vi "LoadImage_Names_more_robust.vi"(11 "Sample Image":path=path "E:/Temp/36ntATgel_20uM_10mMMg_20mMTris_4th/im__000015.tif") -> (1 "Paths":path[](array[path])=[path "E:/Temp/36ntATgel_20uM_10mMMg_20mMTris_4th/im__000003.tif", path "E:/Temp/36ntATgel_20uM_10mMMg_20mMTris_4th/im__000007.tif", path "E:/Temp/36ntATgel_20uM_10mMMg_20mMTris_4th/im__000011.tif", path "E:/Temp/36ntATgel_20uM_10mMMg_20mMTris_4th/im__000015.tif", path "E:/Temp/36ntATgel_20uM_10mMMg_20mMTris_4th/im__000019.tif", path "E:/Temp/36ntATgel_20uM_10mMMg_20mMTris_4th/im__000023.tif", path "E:/Temp/36ntATgel_20uM_10mMMg_20mMTris_4th/im__000027.tif", path "E:/Temp/36ntATgel_20uM_10mMMg_20mMTris_4th/im__000031.tif", path "E:/Temp/36ntATgel_20uM_10mMMg_20mMTris_4th/im__000035.tif", path "E:/Temp/36ntATgel_20uM_10mMMg_20mMTris_4th/im__000039.tif", path "E:/Temp/36ntATgel_20uM_10mMMg_20mMTris_4th/im__000043.tif", path "E:/Temp/36ntATgel_20uM_10mMMg_20mMTris_4th/im__000047.tif", path "E:/Temp/36ntATgel_20uM_10mMMg_20mMTris_4th/im__000051.tif", path "E:/Temp/36ntATgel_20uM_10mMMg_20mMTris_4th/im__000055.tif", path "E:/Temp/36ntATgel_20uM_10mMMg_20mMTris_4th/im__000059.tif", path "E:/Temp/36ntATgel_20uM_10mMMg_20mMTris_4th/im__000063.tif", path "E:/Temp/36ntATgel_20uM_10mMMg_20mMTris_4th/im__000067.tif", path "E:/Temp/36ntATgel_20uM_10mMMg_20mMTris_4th/im__000071.tif", path "E:/Temp/36ntATgel_20uM_10mMMg_20mMTris_4th/im__000075.tif", path "E:/Temp/36ntATgel_20uM_10mMMg_20mMTris_4th/im__000079.tif", path "E:/Temp/36ntATgel_20uM_10mMMg_20mMTris_4th/im__000083.tif", path "E:/Temp/36ntATgel_20uM_10mMMg_20mMTris_4th/im__000087.tif", path "E:/Temp/36ntATgel_20uM_10mMMg_20mMTris_4th/im__000091.tif", path "E:/Temp/36ntATgel_20uM_10mMMg_20mMTris_4th/im__000095.tif", path "E:/Temp/36ntATgel_20uM_10mMMg_20mMTris_4th/im__000099.tif", path "E:/Temp/36ntATgel_20uM_10mMMg_20mMTris_4th/im__000103.tif", path "E:/Temp/36ntATgel_20uM_10mMMg_20mMTris_4th/im__000107.tif", path "E:/Temp/36ntATgel_20uM_10mMMg_20mMTris_4th/im__000111.tif", path "E:/Temp/36ntATgel_20uM_10mMMg_20mMTris_4th/im__000115.tif", path "E:/Temp/36ntATgel_20uM_10mMMg_20mMTris_4th/im__000119.tif", path "E:/Temp/36ntATgel_20uM_10mMMg_20mMTris_4th/im__000123.tif", path "E:/Temp/36ntATgel_20uM_10mMMg_20mMTris_4th/im__000127.tif", path "E:/Temp/36ntATgel_20uM_10mMMg_20mMTris_4th/im__000131.tif", path "E:/Temp/36ntATgel_20uM_10mMMg_20mMTris_4th/im__000135.tif", path "E:/Temp/36ntATgel_20uM_10mMMg_20mMTris_4th/im__000139.tif", path "E:/Temp/36ntATgel_20uM_10mMMg_20mMTris_4th/im__000143.tif", path "E:/Temp/36ntATgel_20uM_10mMMg_20mMTris_4th/im__000147.tif", path "E:/Temp/36ntATgel_20uM_10mMMg_20mMTris_4th/im__000151.tif", path "E:/Temp/36ntATgel_20uM_10mMMg_20mMTris_4th/im__000155.tif", path "E:/Temp/36ntATgel_20uM_10mMMg_20mMTris_4th/im__000159.tif", path "E:/Temp/36ntATgel_20uM_10mMMg_20mMTris_4th/im__000163.tif", path "E:/Temp/36ntATgel_20uM_10mMMg_20mMTris_4th/im__000167.tif", path "E:/Temp/36ntATgel_20uM_10mMMg_20mMTris_4th/im__000171.tif", path "E:/Temp/36ntATgel_20uM_10mMMg_20mMTris_4th/im__000175.tif", path "E:/Temp/36ntATgel_20uM_10mMMg_20mMTris_4th/im__000179.tif", path "E:/Temp/36ntATgel_20uM_10mMMg_20mMTris_4th/im__000183.tif", path "E:/Temp/36ntATgel_20uM_10mMMg_20mMTris_4th/im__000187.tif", path "E:/Temp/36ntATgel_20uM_10mMMg_20mMTris_4th/im__000191.tif", path "E:/Temp/36ntATgel_20uM_10mMMg_20mMTris_4th/im__000195.tif", path "E:/Temp/36ntATgel_20uM_10mMMg_20mMTris_4th/im__000199.tif", path "E:/Temp/36ntATgel_20uM_10mMMg_20mMTris_4th/im__000203.tif", path "E:/Temp/36ntATgel_20uM_10mMMg_20mMTris_4th/im__000207.tif", path "E:/Temp/36ntATgel_20uM_10mMMg_20mMTris_4th/im__000211.tif", path "E:/Temp/36ntATgel_20uM_10mMMg_20mMTris_4th/im__000215.tif", path "E:/Temp/36ntATgel_20uM_10mMMg_20mMTris_4th/im__000219.tif", path "E:/Temp/36ntATgel_20uM_10mMMg_20mMTris_4th/im__000223.tif", path "E:/Temp/36ntATgel_20uM_10mMMg_20mMTris_4th/im__000227.tif", path "E:/Temp/36ntATgel_20uM_10mMMg_20mMTris_4th/im__000231.tif", path "E:/Temp/36ntATgel_20uM_10mMMg_20mMTris_4th/im__000235.tif", path "E:/Temp/36ntATgel_20uM_10mMMg_20mMTris_4th/im__000239.tif", path "E:/Temp/36ntATgel_20uM_10mMMg_20mMTris_4th/im__000243.tif", path "E:/Temp/36ntATgel_20uM_10mMMg_20mMTris_4th/im__000247.tif", path "E:/Temp/36ntATgel_20uM_10mMMg_20mMTris_4th/im__000251.tif", path "E:/Temp/36ntATgel_20uM_10mMMg_20mMTris_4th/im__000255.tif", path "E:/Temp/36ntATgel_20uM_10mMMg_20mMTris_4th/im__000259.tif", path "E:/Temp/36ntATgel_20uM_10mMMg_20mMTris_4th/im__000263.tif", path "E:/Temp/36ntATgel_20uM_10mMMg_20mMTris_4th/im__000267.tif", path "E:/Temp/36ntATgel_20uM_10mMMg_20mMTris_4th/im__000271.tif", path "E:/Temp/36ntATgel_20uM_10mMMg_20mMTris_4th/im__000275.tif", path "E:/Temp/36ntATgel_20uM_10mMMg_20mMTris_4th/im__000279.tif", path "E:/Temp/36ntATgel_20uM_10mMMg_20mMTris_4th/im__000283.tif", path "E:/Temp/36ntATgel_20uM_10mMMg_20mMTris_4th/im__000287.tif", path "E:/Temp/36ntATgel_20uM_10mMMg_20mMTris_4th/im__000291.tif", path "E:/Temp/36ntATgel_20uM_10mMMg_20mMTris_4th/im__000295.tif", path "E:/Temp/36ntATgel_20uM_10mMMg_20mMTris_4th/im__000299.tif", path "E:/Temp/36ntATgel_20uM_10mMMg_20mMTris_4th/im__000303.tif", path "E:/Temp/36ntATgel_20uM_10mMMg_20mMTris_4th/im__000307.tif", path "E:/Temp/36ntATgel_20uM_10mMMg_20mMTris_4th/im__000311.tif", path "E:/Temp/36ntATgel_20uM_10mMMg_20mMTris_4th/im__000315.tif", path "E:/Temp/36ntATgel_20uM_10mMMg_20mMTris_4th/im__000319.tif", path "E:/Temp/36ntATgel_20uM_10mMMg_20mMTris_4th/im__000323.tif", path "E:/Temp/36ntATgel_20uM_10mMMg_20mMTris_4th/im__000327.tif", path "E:/Temp/36ntATgel_20uM_10mMMg_20mMTris_4th/im__000331.tif", path "E:/Temp/36ntATgel_20uM_10mMMg_20mMTris_4th/im__000335.tif", path "E:/Temp/36ntATgel_20uM_10mMMg_20mMTris_4th/im__000339.tif", path "E:/Temp/36ntATgel_20uM_10mMMg_20mMTris_4th/im__000343.tif", path "E:/Temp/36ntATgel_20uM_10mMMg_20mMTris_4th/im__000347.tif", path "E:/Temp/36ntATgel_20uM_10mMMg_20mMTris_4th/im__000351.tif", path "E:/Temp/36ntATgel_20uM_10mMMg_20mMTris_4th/im__000355.tif", path "E:/Temp/36ntATgel_20uM_10mMMg_20mMTris_4th/im__000359.tif", path "E:/Temp/36ntATgel_20uM_10mMMg_20mMTris_4th/im__000363.tif", path "E:/Temp/36ntATgel_20uM_10mMMg_20mMTris_4th/im__000367.tif", path "E:/Temp/36ntATgel_20uM_10mMMg_20mMTris_4th/im__000371.tif", path "E:/Temp/36ntATgel_20uM_10mMMg_20mMTris_4th/im__000375.tif", path "E:/Temp/36ntATgel_20uM_10mMMg_20mMTris_4th/im__000379.tif", path "E:/Temp/36ntATgel_20uM_10mMMg_20mMTris_4th/im__000383.tif", path "E:/Temp/36ntATgel_20uM_10mMMg_20mMTris_4th/im__000387.tif", path "E:/Temp/36ntATgel_20uM_10mMMg_20mMTris_4th/im__000391.tif", path "E:/Temp/36ntATgel_20uM_10mMMg_20mMTris_4th/im__000395.tif", path "E:/Temp/36ntATgel_20uM_10mMMg_20mMTris_4th/im__000399.tif", path "E:/Temp/36ntATgel_20uM_10mMMg_20mMTris_4th/im__000403.tif", path "E:/Temp/36ntATgel_20uM_10mMMg_20mMTris_4th/im__000407.tif", path "E:/Temp/36ntATgel_20uM_10mMMg_20mMTris_4th/im__000411.tif", path "E:/Temp/36ntATgel_20uM_10mMMg_20mMTris_4th/im__000415.tif", path "E:/Temp/36ntATgel_20uM_10mMMg_20mMTris_4th/im__000419.tif", path "E:/Temp/36ntATgel_20uM_10mMMg_20mMTris_4th/im__000423.tif", path "E:/Temp/36ntATgel_20uM_10mMMg_20mMTris_4th/im__000427.tif", path "E:/Temp/36ntATgel_20uM_10mMMg_20mMTris_4th/im__000431.tif", path "E:/Temp/36ntATgel_20uM_10mMMg_20mMTris_4th/im__000435.tif", path "E:/Temp/36ntATgel_20uM_10mMMg_20mMTris_4th/im__000439.tif", path "E:/Temp/36ntATgel_20uM_10mMMg_20mMTris_4th/im__000443.tif", path "E:/Temp/36ntATgel_20uM_10mMMg_20mMTris_4th/im__000447.tif", path "E:/Temp/36ntATgel_20uM_10mMMg_20mMTris_4th/im__000451.tif", path "E:/Temp/36ntATgel_20uM_10mMMg_20mMTris_4th/im__000455.tif", path "E:/Temp/36ntATgel_20uM_10mMMg_20mMTris_4th/im__000459.tif", path "E:/Temp/36ntATgel_20uM_10mMMg_20mMTris_4th/im__000463.tif", path "E:/Temp/36ntATgel_20uM_10mMMg_20mMTris_4th/im__000467.tif", path "E:/Temp/36ntATgel_20uM_10mMMg_20mMTris_4th/im__000471.tif", path "E:/Temp/36ntATgel_20uM_10mMMg_20mMTris_4th/im__000475.tif", path "E:/Temp/36ntATgel_20uM_10mMMg_20mMTris_4th/im__000479.tif", path "E:/Temp/36ntATgel_20uM_10mMMg_20mMTris_4th/im__000483.tif", path "E:/Temp/36ntATgel_20uM_10mMMg_20mMTris_4th/im__000487.tif", path "E:/Temp/36ntATgel_20uM_10mMMg_20mMTris_4th/im__000491.tif", path "E:/Temp/36ntATgel_20uM_10mMMg_20mMTris_4th/im__000495.tif", path "E:/Temp/36ntATgel_20uM_10mMMg_20mMTris_4th/im__000499.tif", path "E:/Temp/36ntATgel_20uM_10mMMg_20mMTris_4th/im__000503.tif", path "E:/Temp/36ntATgel_20uM_10mMMg_20mMTris_4th/im__000507.tif", path "E:/Temp/36ntATgel_20uM_10mMMg_20mMTris_4th/im__000511.tif", path "E:/Temp/36ntATgel_20uM_10mMMg_20mMTris_4th/im__000515.tif", path "E:/Temp/36ntATgel_20uM_10mMMg_20mMTris_4th/im__000519.tif", path "E:/Temp/36ntATgel_20uM_10mMMg_20mMTris_4th/im__000523.tif", path "E:/Temp/36ntATgel_20uM_10mMMg_20mMTris_4th/im__000527.tif", path "E:/Temp/36ntATgel_20uM_10mMMg_20mMTris_4th/im__000531.tif", path "E:/Temp/36ntATgel_20uM_10mMMg_20mMTris_4th/im__000535.tif", path "E:/Temp/36ntATgel_20uM_10mMMg_20mMTris_4th/im__000539.tif", path "E:/Temp/36ntATgel_20uM_10mMMg_20mMTris_4th/im__000543.tif", path "E:/Temp/36ntATgel_20uM_10mMMg_20mMTris_4th/im__000547.tif", path "E:/Temp/36ntATgel_20uM_10mMMg_20mMTris_4th/im__000551.tif", path "E:/Temp/36ntATgel_20uM_10mMMg_20mMTris_4th/im__000555.tif", path "E:/Temp/36ntATgel_20uM_10mMMg_20mMTris_4th/im__000559.tif", path "E:/Temp/36ntATgel_20uM_10mMMg_20mMTris_4th/im__000563.tif", path "E:/Temp/36ntATgel_20uM_10mMMg_20mMTris_4th/im__000567.tif", path "E:/Temp/36ntATgel_20uM_10mMMg_20mMTris_4th/im__000571.tif", path "E:/Temp/36ntATgel_20uM_10mMMg_20mMTris_4th/im__000575.tif", path "E:/Temp/36ntATgel_20uM_10mMMg_20mMTris_4th/im__000579.tif", path "E:/Temp/36ntATgel_20uM_10mMMg_20mMTris_4th/im__000583.tif", path "E:/Temp/36ntATgel_20uM_10mMMg_20mMTris_4th/im__000587.tif", path "E:/Temp/36ntATgel_20uM_10mMMg_20mMTris_4th/im__000591.tif", path "E:/Temp/36ntATgel_20uM_10mMMg_20mMTris_4th/im__000595.tif", path "E:/Temp/36ntATgel_20uM_10mMMg_20mMTris_4th/im__000599.tif", path "E:/Temp/36ntATgel_20uM_10mMMg_20mMTris_4th/im__000603.tif", path "E:/Temp/36ntATgel_20uM_10mMMg_20mMTris_4th/im__000607.tif", path "E:/Temp/36ntATgel_20uM_10mMMg_20mMTris_4th/im__000611.tif", path "E:/Temp/36ntATgel_20uM_10mMMg_20mMTris_4th/im__000615.tif", path "E:/Temp/36ntATgel_20uM_10mMMg_20mMTris_4th/im__000619.tif", path "E:/Temp/36ntATgel_20uM_10mMMg_20mMTris_4th/im__000623.tif", path "E:/Temp/36ntATgel_20uM_10mMMg_20mMTris_4th/im__000627.tif", path "E:/Temp/36ntATgel_20uM_10mMMg_20mMTris_4th/im__000631.tif", path "E:/Temp/36ntATgel_20uM_10mMMg_20mMTris_4th/im__000635.tif", path "E:/Temp/36ntATgel_20uM_10mMMg_20mMTris_4th/im__000639.tif", path "E:/Temp/36ntATgel_20uM_10mMMg_20mMTris_4th/im__000643.tif", path "E:/Temp/36ntATgel_20uM_10mMMg_20mMTris_4th/im__000647.tif", path "E:/Temp/36ntATgel_20uM_10mMMg_20mMTris_4th/im__000651.tif", path "E:/Temp/36ntATgel_20uM_10mMMg_20mMTris_4th/im__000655.tif", path "E:/Temp/36ntATgel_20uM_10mMMg_20mMTris_4th/im__000659.tif", path "E:/Temp/36ntATgel_20uM_10mMMg_20mMTris_4th/im__000663.tif", path "E:/Temp/36ntATgel_20uM_10mMMg_20mMTris_4th/im__000667.tif", path "E:/Temp/36ntATgel_20uM_10mMMg_20mMTris_4th/im__000671.tif", path "E:/Temp/36ntATgel_20uM_10mMMg_20mMTris_4th/im__000675.tif", path "E:/Temp/36ntATgel_20uM_10mMMg_20mMTris_4th/im__000679.tif", path "E:/Temp/36ntATgel_20uM_10mMMg_20mMTris_4th/im__000683.tif", path "E:/Temp/36ntATgel_20uM_10mMMg_20mMTris_4th/im__000687.tif", path "E:/Temp/36ntATgel_20uM_10mMMg_20mMTris_4th/im__000691.tif", path "E:/Temp/36ntATgel_20uM_10mMMg_20mMTris_4th/im__000695.tif", path "E:/Temp/36ntATgel_20uM_10mMMg_20mMTris_4th/im__000699.tif", path "E:/Temp/36ntATgel_20uM_10mMMg_20mMTris_4th/im__000703.tif", path "E:/Temp/36ntATgel_20uM_10mMMg_20mMTris_4th/im__000707.tif", path "E:/Temp/36ntATgel_20uM_10mMMg_20mMTris_4th/im__000711.tif", path "E:/Temp/36ntATgel_20uM_10mMMg_20mMTris_4th/im__000715.tif", path "E:/Temp/36ntATgel_20uM_10mMMg_20mMTris_4th/im__000719.tif", path "E:/Temp/36ntATgel_20uM_10mMMg_20mMTris_4th/im__000723.tif", path "E:/Temp/36ntATgel_20uM_10mMMg_20mMTris_4th/im__000727.tif", path "E:/Temp/36ntATgel_20uM_10mMMg_20mMTris_4th/im__000731.tif", path "E:/Temp/36ntATgel_20uM_10mMMg_20mMTris_4th/im__000735.tif", path "E:/Temp/36ntATgel_20uM_10mMMg_20mMTris_4th/im__000739.tif", path "E:/Temp/36ntATgel_20uM_10mMMg_20mMTris_4th/im__000743.tif", path "E:/Temp/36ntATgel_20uM_10mMMg_20mMTris_4th/im__000747.tif", path "E:/Temp/36ntATgel_20uM_10mMMg_20mMTris_4th/im__000751.tif", path "E:/Temp/36ntATgel_20uM_10mMMg_20mMTris_4th/im__000755.tif", path "E:/Temp/36ntATgel_20uM_10mMMg_20mMTris_4th/im__000759.tif", path "E:/Temp/36ntATgel_20uM_10mMMg_20mMTris_4th/im__000763.tif", path "E:/Temp/36ntATgel_20uM_10mMMg_20mMTris_4th/im__000767.tif", path "E:/Temp/36ntATgel_20uM_10mMMg_20mMTris_4th/im__000771.tif", path "E:/Temp/36ntATgel_20uM_10mMMg_20mMTris_4th/im__000775.tif", path "E:/Temp/36ntATgel_20uM_10mMMg_20mMTris_4th/im__000779.tif", path "E:/Temp/36ntATgel_20uM_10mMMg_20mMTris_4th/im__000783.tif", path "E:/Temp/36ntATgel_20uM_10mMMg_20mMTris_4th/im__000787.tif", path "E:/Temp/36ntATgel_20uM_10mMMg_20mMTris_4th/im__000791.tif", path "E:/Temp/36ntATgel_20uM_10mMMg_20mMTris_4th/im__000795.tif", path "E:/Temp/36ntATgel_20uM_10mMMg_20mMTris_4th/im__000799.tif", path "E:/Temp/36ntATgel_20uM_10mMMg_20mMTris_4th/im__000803.tif", path "E:/Temp/36ntATgel_20uM_10mMMg_20mMTris_4th/im__000807.tif", path "E:/Temp/36ntATgel_20uM_10mMMg_20mMTris_4th/im__000811.tif", path "E:/Temp/36ntATgel_20uM_10mMMg_20mMTris_4th/im__000815.tif", path "E:/Temp/36ntATgel_20uM_10mMMg_20mMTris_4th/im__000819.tif", path "E:/Temp/36ntATgel_20uM_10mMMg_20mMTris_4th/im__000823.tif", path "E:/Temp/36ntATgel_20uM_10mMMg_20mMTris_4th/im__000827.tif", path "E:/Temp/36ntATgel_20uM_10mMMg_20mMTris_4th/im__000831.tif", path "E:/Temp/36ntATgel_20uM_10mMMg_20mMTris_4th/im__000835.tif", path "E:/Temp/36ntATgel_20uM_10mMMg_20mMTris_4th/im__000839.tif", path "E:/Temp/36ntATgel_20uM_10mMMg_20mMTris_4th/im__000843.tif", path "E:/Temp/36ntATgel_20uM_10mMMg_20mMTris_4th/im__000847.tif", path "E:/Temp/36ntATgel_20uM_10mMMg_20mMTris_4th/im__000851.tif", path "E:/Temp/36ntATgel_20uM_10mMMg_20mMTris_4th/im__000855.tif", path "E:/Temp/36ntATgel_20uM_10mMMg_20mMTris_4th/im__000859.tif", path "E:/Temp/36ntATgel_20uM_10mMMg_20mMTris_4th/im__000863.tif", path "E:/Temp/36ntATgel_20uM_10mMMg_20mMTris_4th/im__000867.tif", path "E:/Temp/36ntATgel_20uM_10mMMg_20mMTris_4th/im__000871.tif", path "E:/Temp/36ntATgel_20uM_10mMMg_20mMTris_4th/im__000875.tif", path "E:/Temp/36ntATgel_20uM_10mMMg_20mMTris_4th/im__000879.tif", path "E:/Temp/36ntATgel_20uM_10mMMg_20mMTris_4th/im__000883.tif", path "E:/Temp/36ntATgel_20uM_10mMMg_20mMTris_4th/im__000887.tif", path "E:/Temp/36ntATgel_20uM_10mMMg_20mMTris_4th/im__000891.tif", path "E:/Temp/36ntATgel_20uM_10mMMg_20mMTris_4th/im__000895.tif", path "E:/Temp/36ntATgel_20uM_10mMMg_20mMTris_4th/im__000899.tif", path "E:/Temp/36ntATgel_20uM_10mMMg_20mMTris_4th/im__000903.tif", path "E:/Temp/36ntATgel_20uM_10mMMg_20mMTris_4th/im__000907.tif", path "E:/Temp/36ntATgel_20uM_10mMMg_20mMTris_4th/im__000911.tif", path "E:/Temp/36ntATgel_20uM_10mMMg_20mMTris_4th/im__000915.tif", path "E:/Temp/36ntATgel_20uM_10mMMg_20mMTris_4th/im__000919.tif", path "E:/Temp/36ntATgel_20uM_10mMMg_20mMTris_4th/im__000923.tif", path "E:/Temp/36ntATgel_20uM_10mMMg_20mMTris_4th/im__000927.tif", path "E:/Temp/36ntATgel_20uM_10mMMg_20mMTris_4th/im__000931.tif", path "E:/Temp/36ntATgel_20uM_10mMMg_20mMTris_4th/im__000935.tif", path "E:/Temp/36ntATgel_20uM_10mMMg_20mMTris_4th/im__000939.tif", path "E:/Temp/36ntATgel_20uM_10mMMg_20mMTris_4th/im__000943.tif", path "E:/Temp/36ntATgel_20uM_10mMMg_20mMTris_4th/im__000947.tif", path "E:/Temp/36ntATgel_20uM_10mMMg_20mMTris_4th/im__000951.tif", path "E:/Temp/36ntATgel_20uM_10mMMg_20mMTris_4th/im__000955.tif", path "E:/Temp/36ntATgel_20uM_10mMMg_20mMTris_4th/im__000959.tif", path "E:/Temp/36ntATgel_20uM_10mMMg_20mMTris_4th/im__000963.tif", path "E:/Temp/36ntATgel_20uM_10mMMg_20mMTris_4th/im__000967.tif", path "E:/Temp/36ntATgel_20uM_10mMMg_20mMTris_4th/im__000971.tif", path "E:/Temp/36ntATgel_20uM_10mMMg_20mMTris_4th/im__000975.tif", path "E:/Temp/36ntATgel_20uM_10mMMg_20mMTris_4th/im__000979.tif", path "E:/Temp/36ntATgel_20uM_10mMMg_20mMTris_4th/im__000983.tif", path "E:/Temp/36ntATgel_20uM_10mMMg_20mMTris_4th/im__000987.tif", path "E:/Temp/36ntATgel_20uM_10mMMg_20mMTris_4th/im__000991.tif", path "E:/Temp/36ntATgel_20uM_10mMMg_20mMTris_4th/im__000995.tif", path "E:/Temp/36ntATgel_20uM_10mMMg_20mMTris_4th/im__000999.tif", path "E:/Temp/36ntATgel_20uM_10mMMg_20mMTris_4th/im__001003.tif", path "E:/Temp/36ntATgel_20uM_10mMMg_20mMTris_4th/im__001007.tif", path "E:/Temp/36ntATgel_20uM_10mMMg_20mMTris_4th/im__001011.tif", path "E:/Temp/36ntATgel_20uM_10mMMg_20mMTris_4th/im__001015.tif", path "E:/Temp/36ntATgel_20uM_10mMMg_20mMTris_4th/im__001019.tif", path "E:/Temp/36ntATgel_20uM_10mMMg_20mMTris_4th/im__001023.tif", path "E:/Temp/36ntATgel_20uM_10mMMg_20mMTris_4th/im__001027.tif", path "E:/Temp/36ntATgel_20uM_10mMMg_20mMTris_4th/im__001031.tif", path "E:/Temp/36ntATgel_20uM_10mMMg_20mMTris_4th/im__001035.tif", path "E:/Temp/36ntATgel_20uM_10mMMg_20mMTris_4th/im__001039.tif", path "E:/Temp/36ntATgel_20uM_10mMMg_20mMTris_4th/im__001043.tif", path "E:/Temp/36ntATgel_20uM_10mMMg_20mMTris_4th/im__001047.tif", path "E:/Temp/36ntATgel_20uM_10mMMg_20mMTris_4th/im__001051.tif", path "E:/Temp/36ntATgel_20uM_10mMMg_20mMTris_4th/im__001055.tif", path "E:/Temp/36ntATgel_20uM_10mMMg_20mMTris_4th/im__001059.tif", path "E:/Temp/36ntATgel_20uM_10mMMg_20mMTris_4th/im__001063.tif", path "E:/Temp/36ntATgel_20uM_10mMMg_20mMTris_4th/im__001067.tif", path "E:/Temp/36ntATgel_20uM_10mMMg_20mMTris_4th/im__001071.tif", path "E:/Temp/36ntATgel_20uM_10mMMg_20mMTris_4th/im__001075.tif", path "E:/Temp/36ntATgel_20uM_10mMMg_20mMTris_4th/im__001079.tif", path "E:/Temp/36ntATgel_20uM_10mMMg_20mMTris_4th/im__001083.tif", path "E:/Temp/36ntATgel_20uM_10mMMg_20mMTris_4th/im__001087.tif", path "E:/Temp/36ntATgel_20uM_10mMMg_20mMTris_4th/im__001091.tif", path "E:/Temp/36ntATgel_20uM_10mMMg_20mMTris_4th/im__001095.tif", path "E:/Temp/36ntATgel_20uM_10mMMg_20mMTris_4th/im__001099.tif", path "E:/Temp/36ntATgel_20uM_10mMMg_20mMTris_4th/im__001103.tif", path "E:/Temp/36ntATgel_20uM_10mMMg_20mMTris_4th/im__001107.tif", path "E:/Temp/36ntATgel_20uM_10mMMg_20mMTris_4th/im__001111.tif", path "E:/Temp/36ntATgel_20uM_10mMMg_20mMTris_4th/im__001115.tif", path "E:/Temp/36ntATgel_20uM_10mMMg_20mMTris_4th/im__001119.tif", path "E:/Temp/36ntATgel_20uM_10mMMg_20mMTris_4th/im__001123.tif", path "E:/Temp/36ntATgel_20uM_10mMMg_20mMTris_4th/im__001127.tif", path "E:/Temp/36ntATgel_20uM_10mMMg_20mMTris_4th/im__001131.tif", path "E:/Temp/36ntATgel_20uM_10mMMg_20mMTris_4th/im__001135.tif", path "E:/Temp/36ntATgel_20uM_10mMMg_20mMTris_4th/im__001139.tif", path "E:/Temp/36ntATgel_20uM_10mMMg_20mMTris_4th/im__001143.tif", path "E:/Temp/36ntATgel_20uM_10mMMg_20mMTris_4th/im__001147.tif", path "E:/Temp/36ntATgel_20uM_10mMMg_20mMTris_4th/im__001151.tif", path "E:/Temp/36ntATgel_20uM_10mMMg_20mMTris_4th/im__001155.tif", path "E:/Temp/36ntATgel_20uM_10mMMg_20mMTris_4th/im__001159.tif", path "E:/Temp/36ntATgel_20uM_10mMMg_20mMTris_4th/im__001163.tif", path "E:/Temp/36ntATgel_20uM_10mMMg_20mMTris_4th/im__001167.tif", path "E:/Temp/36ntATgel_20uM_10mMMg_20mMTris_4th/im__001171.tif", path "E:/Temp/36ntATgel_20uM_10mMMg_20mMTris_4th/im__001175.tif", path "E:/Temp/36ntATgel_20uM_10mMMg_20mMTris_4th/im__001179.tif", path "E:/Temp/36ntATgel_20uM_10mMMg_20mMTris_4th/im__001183.tif", path "E:/Temp/36ntATgel_20uM_10mMMg_20mMTris_4th/im__001187.tif", path "E:/Temp/36ntATgel_20uM_10mMMg_20mMTris_4th/im__001191.tif", path "E:/Temp/36ntATgel_20uM_10mMMg_20mMTris_4th/im__001195.tif", path "E:/Temp/36ntATgel_20uM_10mMMg_20mMTris_4th/im__001199.tif", path "E:/Temp/36ntATgel_20uM_10mMMg_20mMTris_4th/im__001203.tif", path "E:/Temp/36ntATgel_20uM_10mMMg_20mMTris_4th/im__001207.tif", path "E:/Temp/36ntATgel_20uM_10mMMg_20mMTris_4th/im__001211.tif", path "E:/Temp/36ntATgel_20uM_10mMMg_20mMTris_4th/im__001215.tif", path "E:/Temp/36ntATgel_20uM_10mMMg_20mMTris_4th/im__001219.tif", path "E:/Temp/36ntATgel_20uM_10mMMg_20mMTris_4th/im__001223.tif", path "E:/Temp/36ntATgel_20uM_10mMMg_20mMTris_4th/im__001227.tif", path "E:/Temp/36ntATgel_20uM_10mMMg_20mMTris_4th/im__001231.tif", path "E:/Temp/36ntATgel_20uM_10mMMg_20mMTris_4th/im__001235.tif", path "E:/Temp/36ntATgel_20uM_10mMMg_20mMTris_4th/im__001239.tif", path "E:/Temp/36ntATgel_20uM_10mMMg_20mMTris_4th/im__001243.tif", path "E:/Temp/36ntATgel_20uM_10mMMg_20mMTris_4th/im__001247.tif", path "E:/Temp/36ntATgel_20uM_10mMMg_20mMTris_4th/im__001251.tif", path "E:/Temp/36ntATgel_20uM_10mMMg_20mMTris_4th/im__001255.tif", path "E:/Temp/36ntATgel_20uM_10mMMg_20mMTris_4th/im__001259.tif", path "E:/Temp/36ntATgel_20uM_10mMMg_20mMTris_4th/im__001263.tif", path "E:/Temp/36ntATgel_20uM_10mMMg_20mMTris_4th/im__001267.tif", path "E:/Temp/36ntATgel_20uM_10mMMg_20mMTris_4th/im__001271.tif", path "E:/Temp/36ntATgel_20uM_10mMMg_20mMTris_4th/im__001275.tif", path "E:/Temp/36ntATgel_20uM_10mMMg_20mMTris_4th/im__001279.tif", path "E:/Temp/36ntATgel_20uM_10mMMg_20mMTris_4th/im__001283.tif", path "E:/Temp/36ntATgel_20uM_10mMMg_20mMTris_4th/im__001287.tif", path "E:/Temp/36ntATgel_20uM_10mMMg_20mMTris_4th/im__001291.tif", path "E:/Temp/36ntATgel_20uM_10mMMg_20mMTris_4th/im__001295.tif", path "E:/Temp/36ntATgel_20uM_10mMMg_20mMTris_4th/im__001299.tif", path "E:/Temp/36ntATgel_20uM_10mMMg_20mMTris_4th/im__001303.tif", path "E:/Temp/36ntATgel_20uM_10mMMg_20mMTris_4th/im__001307.tif", path "E:/Temp/36ntATgel_20uM_10mMMg_20mMTris_4th/im__001311.tif", path "E:/Temp/36ntATgel_20uM_10mMMg_20mMTris_4th/im__001315.tif", path "E:/Temp/36ntATgel_20uM_10mMMg_20mMTris_4th/im__001319.tif", path "E:/Temp/36ntATgel_20uM_10mMMg_20mMTris_4th/im__001323.tif", path "E:/Temp/36ntATgel_20uM_10mMMg_20mMTris_4th/im__001327.tif", path "E:/Temp/36ntATgel_20uM_10mMMg_20mMTris_4th/im__001331.tif", path "E:/Temp/36ntATgel_20uM_10mMMg_20mMTris_4th/im__001335.tif", path "E:/Temp/36ntATgel_20uM_10mMMg_20mMTris_4th/im__001339.tif", path "E:/Temp/36ntATgel_20uM_10mMMg_20mMTris_4th/im__001343.tif", path "E:/Temp/36ntATgel_20uM_10mMMg_20mMTris_4th/im__001347.tif", path "E:/Temp/36ntATgel_20uM_10mMMg_20mMTris_4th/im__001351.tif", path "E:/Temp/36ntATgel_20uM_10mMMg_20mMTris_4th/im__001355.tif", path "E:/Temp/36ntATgel_20uM_10mMMg_20mMTris_4th/im__001359.tif", path "E:/Temp/36ntATgel_20uM_10mMMg_20mMTris_4th/im__001363.tif", path "E:/Temp/36ntATgel_20uM_10mMMg_20mMTris_4th/im__001367.tif", path "E:/Temp/36ntATgel_20uM_10mMMg_20mMTris_4th/im__001371.tif", path "E:/Temp/36ntATgel_20uM_10mMMg_20mMTris_4th/im__001375.tif", path "E:/Temp/36ntATgel_20uM_10mMMg_20mMTris_4th/im__001379.tif", path "E:/Temp/36ntATgel_20uM_10mMMg_20mMTris_4th/im__001383.tif", path "E:/Temp/36ntATgel_20uM_10mMMg_20mMTris_4th/im__001387.tif", path "E:/Temp/36ntATgel_20uM_10mMMg_20mMTris_4th/im__001391.tif", path "E:/Temp/36ntATgel_20uM_10mMMg_20mMTris_4th/im__001395.tif", path "E:/Temp/36ntATgel_20uM_10mMMg_20mMTris_4th/im__001399.tif", path "E:/Temp/36ntATgel_20uM_10mMMg_20mMTris_4th/im__001403.tif", path "E:/Temp/36ntATgel_20uM_10mMMg_20mMTris_4th/im__001407.tif", path "E:/Temp/36ntATgel_20uM_10mMMg_20mMTris_4th/im__001411.tif", path "E:/Temp/36ntATgel_20uM_10mMMg_20mMTris_4th/im__001415.tif", path "E:/Temp/36ntATgel_20uM_10mMMg_20mMTris_4th/im__001419.tif", path "E:/Temp/36ntATgel_20uM_10mMMg_20mMTris_4th/im__001423.tif", path "E:/Temp/36ntATgel_20uM_10mMMg_20mMTris_4th/im__001427.tif", path "E:/Temp/36ntATgel_20uM_10mMMg_20mMTris_4th/im__001431.tif", path "E:/Temp/36ntATgel_20uM_10mMMg_20mMTris_4th/im__001435.tif", path "E:/Temp/36ntATgel_20uM_10mMMg_20mMTris_4th/im__001439.tif", path "E:/Temp/36ntATgel_20uM_10mMMg_20mMTris_4th/im__001443.tif", path "E:/Temp/36ntATgel_20uM_10mMMg_20mMTris_4th/im__001447.tif", path "E:/Temp/36ntATgel_20uM_10mMMg_20mMTris_4th/im__001451.tif", path "E:/Temp/36ntATgel_20uM_10mMMg_20mMTris_4th/im__001455.tif", path "E:/Temp/36ntATgel_20uM_10mMMg_20mMTris_4th/im__001459.tif", path "E:/Temp/36ntATgel_20uM_10mMMg_20mMTris_4th/im__001463.tif", path "E:/Temp/36ntATgel_20uM_10mMMg_20mMTris_4th/im__001467.tif", path "E:/Temp/36ntATgel_20uM_10mMMg_20mMTris_4th/im__001471.tif", path "E:/Temp/36ntATgel_20uM_10mMMg_20mMTris_4th/im__001475.tif", path "E:/Temp/36ntATgel_20uM_10mMMg_20mMTris_4th/im__001479.tif", path "E:/Temp/36ntATgel_20uM_10mMMg_20mMTris_4th/im__001483.tif", path "E:/Temp/36ntATgel_20uM_10mMMg_20mMTris_4th/im__001487.tif", path "E:/Temp/36ntATgel_20uM_10mMMg_20mMTris_4th/im__001491.tif", path "E:/Temp/36ntATgel_20uM_10mMMg_20mMTris_4th/im__001495.tif", path "E:/Temp/36ntATgel_20uM_10mMMg_20mMTris_4th/im__001499.tif", path "E:/Temp/36ntATgel_20uM_10mMMg_20mMTris_4th/im__001503.tif", path "E:/Temp/36ntATgel_20uM_10mMMg_20mMTris_4th/im__001507.tif", path "E:/Temp/36ntATgel_20uM_10mMMg_20mMTris_4th/im__001511.tif", path "E:/Temp/36ntATgel_20uM_10mMMg_20mMTris_4th/im__001515.tif", path "E:/Temp/36ntATgel_20uM_10mMMg_20mMTris_4th/im__001519.tif", path "E:/Temp/36ntATgel_20uM_10mMMg_20mMTris_4th/im__001523.tif", path "E:/Temp/36ntATgel_20uM_10mMMg_20mMTris_4th/im__001527.tif", path "E:/Temp/36ntATgel_20uM_10mMMg_20mMTris_4th/im__001531.tif", path "E:/Temp/36ntATgel_20uM_10mMMg_20mMTris_4th/im__001535.tif", path "E:/Temp/36ntATgel_20uM_10mMMg_20mMTris_4th/im__001539.tif", path "E:/Temp/36ntATgel_20uM_10mMMg_20mMTris_4th/im__001543.tif", path "E:/Temp/36ntATgel_20uM_10mMMg_20mMTris_4th/im__001547.tif", path "E:/Temp/36ntATgel_20uM_10mMMg_20mMTris_4th/im__001551.tif", path "E:/Temp/36ntATgel_20uM_10mMMg_20mMTris_4th/im__001555.tif", path "E:/Temp/36ntATgel_20uM_10mMMg_20mMTris_4th/im__001559.tif", path "E:/Temp/36ntATgel_20uM_10mMMg_20mMTris_4th/im__001563.tif", path "E:/Temp/36ntATgel_20uM_10mMMg_20mMTris_4th/im__001567.tif", path "E:/Temp/36ntATgel_20uM_10mMMg_20mMTris_4th/im__001571.tif", path "E:/Temp/36ntATgel_20uM_10mMMg_20mMTris_4th/im__001575.tif", path "E:/Temp/36ntATgel_20uM_10mMMg_20mMTris_4th/im__001579.tif", path "E:/Temp/36ntATgel_20uM_10mMMg_20mMTris_4th/im__001583.tif", path "E:/Temp/36ntATgel_20uM_10mMMg_20mMTris_4th/im__001587.tif", path "E:/Temp/36ntATgel_20uM_10mMMg_20mMTris_4th/im__001591.tif", path "E:/Temp/36ntATgel_20uM_10mMMg_20mMTris_4th/im__001595.tif", path "E:/Temp/36ntATgel_20uM_10mMMg_20mMTris_4th/im__001599.tif", path "E:/Temp/36ntATgel_20uM_10mMMg_20mMTris_4th/im__001603.tif", path "E:/Temp/36ntATgel_20uM_10mMMg_20mMTris_4th/im__001607.tif", path "E:/Temp/36ntATgel_20uM_10mMMg_20mMTris_4th/im__001611.tif", path "E:/Temp/36ntATgel_20uM_10mMMg_20mMTris_4th/im__001615.tif", path "E:/Temp/36ntATgel_20uM_10mMMg_20mMTris_4th/im__001619.tif", path "E:/Temp/36ntATgel_20uM_10mMMg_20mMTris_4th/im__001623.tif", path "E:/Temp/36ntATgel_20uM_10mMMg_20mMTris_4th/im__001627.tif", path "E:/Temp/36ntATgel_20uM_10mMMg_20mMTris_4th/im__001631.tif", path "E:/Temp/36ntATgel_20uM_10mMMg_20mMTris_4th/im__001635.tif", path "E:/Temp/36ntATgel_20uM_10mMMg_20mMTris_4th/im__001639.tif", path "E:/Temp/36ntATgel_20uM_10mMMg_20mMTris_4th/im__001643.tif", path "E:/Temp/36ntATgel_20uM_10mMMg_20mMTris_4th/im__001647.tif", path "E:/Temp/36ntATgel_20uM_10mMMg_20mMTris_4th/im__001651.tif", path "E:/Temp/36ntATgel_20uM_10mMMg_20mMTris_4th/im__001655.tif", path "E:/Temp/36ntATgel_20uM_10mMMg_20mMTris_4th/im__001659.tif", path "E:/Temp/36ntATgel_20uM_10mMMg_20mMTris_4th/im__001663.tif", path "E:/Temp/36ntATgel_20uM_10mMMg_20mMTris_4th/im__001667.tif", path "E:/Temp/36ntATgel_20uM_10mMMg_20mMTris_4th/im__001671.tif", path "E:/Temp/36ntATgel_20uM_10mMMg_20mMTris_4th/im__001675.tif", path "E:/Temp/36ntATgel_20uM_10mMMg_20mMTris_4th/im__001679.tif", path "E:/Temp/36ntATgel_20uM_10mMMg_20mMTris_4th/im__001683.tif", path "E:/Temp/36ntATgel_20uM_10mMMg_20mMTris_4th/im__001687.tif", path "E:/Temp/36ntATgel_20uM_10mMMg_20mMTris_4th/im__001691.tif", path "E:/Temp/36ntATgel_20uM_10mMMg_20mMTris_4th/im__001695.tif", path "E:/Temp/36ntATgel_20uM_10mMMg_20mMTris_4th/im__001699.tif", path "E:/Temp/36ntATgel_20uM_10mMMg_20mMTris_4th/im__001703.tif", path "E:/Temp/36ntATgel_20uM_10mMMg_20mMTris_4th/im__001707.tif", path "E:/Temp/36ntATgel_20uM_10mMMg_20mMTris_4th/im__001711.tif", path "E:/Temp/36ntATgel_20uM_10mMMg_20mMTris_4th/im__001715.tif", path "E:/Temp/36ntATgel_20uM_10mMMg_20mMTris_4th/im__001719.tif", path "E:/Temp/36ntATgel_20uM_10mMMg_20mMTris_4th/im__001723.tif", path "E:/Temp/36ntATgel_20uM_10mMMg_20mMTris_4th/im__001727.tif", path "E:/Temp/36ntATgel_20uM_10mMMg_20mMTris_4th/im__001731.tif", path "E:/Temp/36ntATgel_20uM_10mMMg_20mMTris_4th/im__001735.tif", path "E:/Temp/36ntATgel_20uM_10mMMg_20mMTris_4th/im__001739.tif", path "E:/Temp/36ntATgel_20uM_10mMMg_20mMTris_4th/im__001743.tif", path "E:/Temp/36ntATgel_20uM_10mMMg_20mMTris_4th/im__001747.tif", path "E:/Temp/36ntATgel_20uM_10mMMg_20mMTris_4th/im__001751.tif", path "E:/Temp/36ntATgel_20uM_10mMMg_20mMTris_4th/im__001755.tif", path "E:/Temp/36ntATgel_20uM_10mMMg_20mMTris_4th/im__001759.tif", path "E:/Temp/36ntATgel_20uM_10mMMg_20mMTris_4th/im__001763.tif", path "E:/Temp/36ntATgel_20uM_10mMMg_20mMTris_4th/im__001767.tif", path "E:/Temp/36ntATgel_20uM_10mMMg_20mMTris_4th/im__001771.tif", path "E:/Temp/36ntATgel_20uM_10mMMg_20mMTris_4th/im__001775.tif"], 3 "Film length":i32=444)   [LabVIEW 2014]
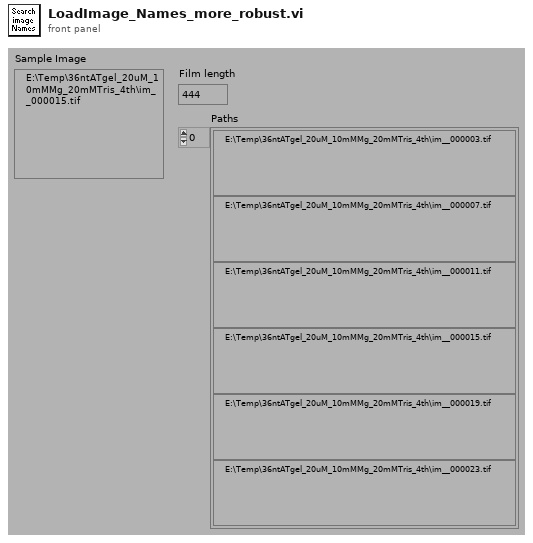
[diagram p1: front panel]
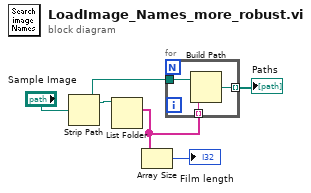
[diagram p0: block diagram]
diagram:
  n1 = Strip Path(path="Sample Image") -> (stripped path=w3:path)  [unwired: 1 out]
  n2 = List Folder(path=w3) -> (filenames=w2:string[])  [unwired: 3 in, 3 out]
  n3 = Array Size(array=w2) -> (size(s)=→"Film length":i32)
  n4 = for {
    tunnel: w3 -> [w8]
    tunnel: w2 -> [w7] mode=indexing
    tunnel: [w6] -> w1 mode=indexing
    n5 = Build Path(base path=w8, name or relative path=w7) -> (appended path=w6:path)
  }
  "Paths" <- w1
